vi "Configure 4W High Accuracy.vi"() -> (15 "error out":errorcluster)   [LabVIEW 2010]
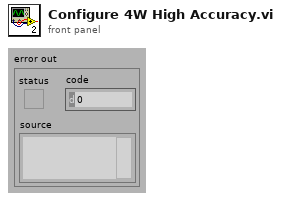
[diagram p1: front panel]
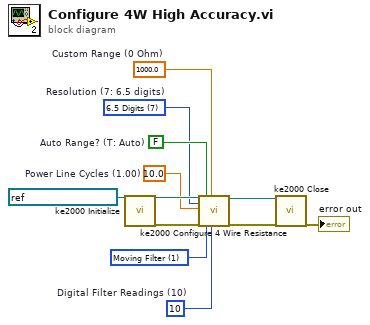
[diagram p0: block diagram]
diagram:
  w1 = u16 7 items=["3.5 Digits"=4, "4.5 Digits"=5, "5.5 Digits"=6, "6.5 Digits"=7]  # Resolution (7: 6.5 digits)
  w2 = 10  # Digital Filter Readings (10)
  w3 = u16 1 items=["Off", "Moving Filter", "Repeating Filter"] ("Digital Filter (0: Off)")
  w5 = 1000.0  # Custom Range (0 Ohm)
  w6 = FALSE  # Auto Range? (T: Auto)
  w7 = 10.0  # Power Line Cycles (1.00)
  n1 = call "ke2000 Initialize.vi"("VISA resource name"=refnum<visa-resource-name> "GPIB0::8::INSTR") -> ("VISA resource name out"=w12:refnum<visa-resource-name>, "error out"=w9:errorcluster)  [unwired: 17 in]
  n2 = call "ke2000 Configure 4 Wire Resistance.vi"("VISA resource name"=w12, "Resolution (7: 6.5 digits)"=w1, "Power Line Cycles (1.00)"=w7, "error in (no error)"=w9, "Auto Range? (T: Auto)"=w6, "Digital Filter (0: Off)"=w3, "Custom Range (0 Ohm)"=w5, "Digital Filter Readings (10)"=w2) -> ("VISA resource name out"=w10:refnum<visa-resource-name>, "error out"=w8:errorcluster)  [unwired: 10 in]
  n3 = call "ke2000 Close.vi"("VISA resource name"=w10, "error in (no error)"=w8) -> ("error out"=→"error out":errorcluster)  [unwired: 17 in]
